vi "Write Buffer to Log Copy.vi"() -> ()   [LabVIEW 2018]
panel:
  out "error out":errorcluster
  in  "error in":errorcluster
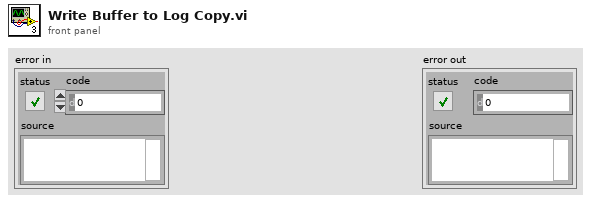
[diagram p1: front panel]
types:
  T1 = typedef "WPI_SerialPortRef.ctl" = cluster{"DevStatus":errorcluster, "Serial Port Name":refnum<visa-resource-name>}
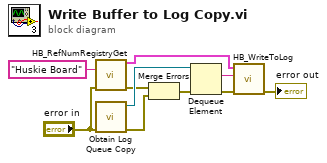
[diagram p0: block diagram]
diagram:
  n1 = call <vilib>:"HB_RefNumRegistryGet.vi"("refnum name"="Huskie Board", "error in (no error)"="error in") -> ("HBDevRef"=w10:T1, "error out"=w5:errorcluster)  [unwired: 12 in]
  n2 = call "Obtain Log Queue Copy.vi"("error in"="error in") -> ("error out"=w4:errorcluster, "queue out"=w8:refnum<queue>)  [unwired: 9 in]
  n3 = Merge Errors(w5, w4) -> (w6:errorcluster)
  n4 = Dequeue Element(queue=w8, error in (no error)=w6) -> (element=w7:string, error out=w3:errorcluster)  [unwired: 1 in, 2 out]
  n5 = call "HB_WriteToLog.vi"("error in (no error)"=w3, "Log string"=w7, "HBDevRef"=w10) -> ("error out"=→"error out":errorcluster)  [unwired: 7 in, 1 out]
